vi "2015 Summary.vi"(8 "error in (no error)":errorcluster, 10 "2015 Cycle Stats":T1, 11 "File Locations":T2) -> (0 "error out":errorcluster)   [LabVIEW 2014]
uses:
  Utility/Save File/Public/Type Definitions/Save File File Paths.ctl
  Type Definitions/2015 Program/2015 Cycle Stats.ctl
  Utility/Save File/Save File.lvlib
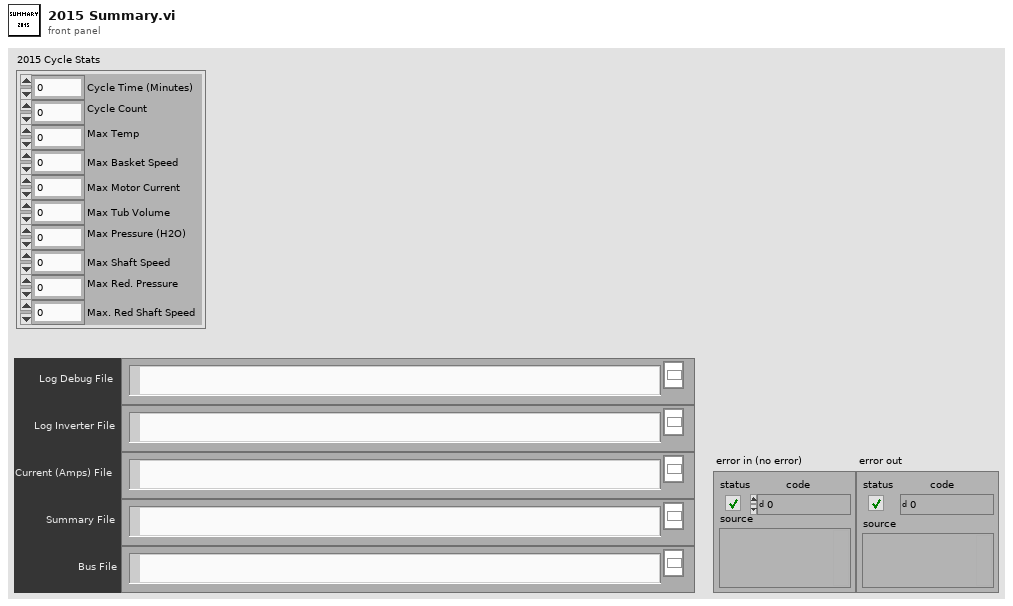
[diagram p1: front panel]
types:
  T1 = typedef "2015 Cycle Stats.ctl" = cluster{"Cycle Time (Minutes)":dbl, "Max Temp":dbl, "Max Basket Speed":dbl, "Max Motor Current":dbl, "Max Tub Volume":dbl, "Max Pressure (H2O)":dbl, "Cycle Count":dbl, "Max Shaft Speed ":dbl, "Max Red. Pressure":dbl, "Max. Red Shaft Speed":dbl}
  T2 = typedef "Save File.lvlib/Save File File Paths.ctl" = cluster{"Log Debug File":path, "Log Inverter File":path, "Summary File":path, "Bus File":path, "Current (Amps) File":path}
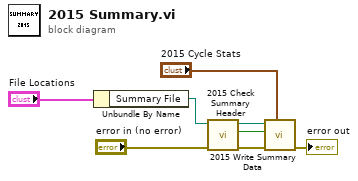
[diagram p0: block diagram]
diagram:
  n1 = Unbundle By Name("File Locations") -> ("Summary File"=w4:path)
  n2 = call "2015 Check Summary Header.vi"("Error In"="error in (no error)", "Summary File"=w4) -> ("Error Out"=w6:errorcluster, "Write Header?"=w1:bool, "Summary Path"=w3:path)  [unwired: 7 in]
  n3 = call "2015 Write Summary Data.vi"("2015 Cycle Stats"="2015 Cycle Stats", "Error In"=w6, "Write Header?"=w1, "new file path (Not A Path if cancelled)"=w3) -> ("Error Out"=→"error out":errorcluster)  [unwired: 7 in]
